vi "test Create Non-default Tag.vi"(8 "error in (no error)":errorcluster, 11 "TestCase in":refnum<class "TagTests.lvclass">) -> (0 "error out":errorcluster, 3 "TestCase out":refnum<class "TagTests.lvclass">)   [LabVIEW 2014, in "TagTests.lvclass"]
uses:
  TagTests.lvclass
  SPLAT/Tag.lvclass
  <vilib>/addons/_JKI Toolkits/VI Tester/TestCase.llb/TestCase.lvclass
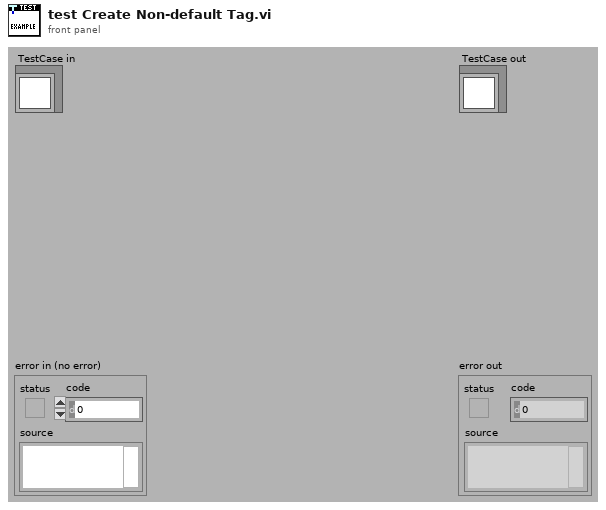
[diagram p1: front panel]
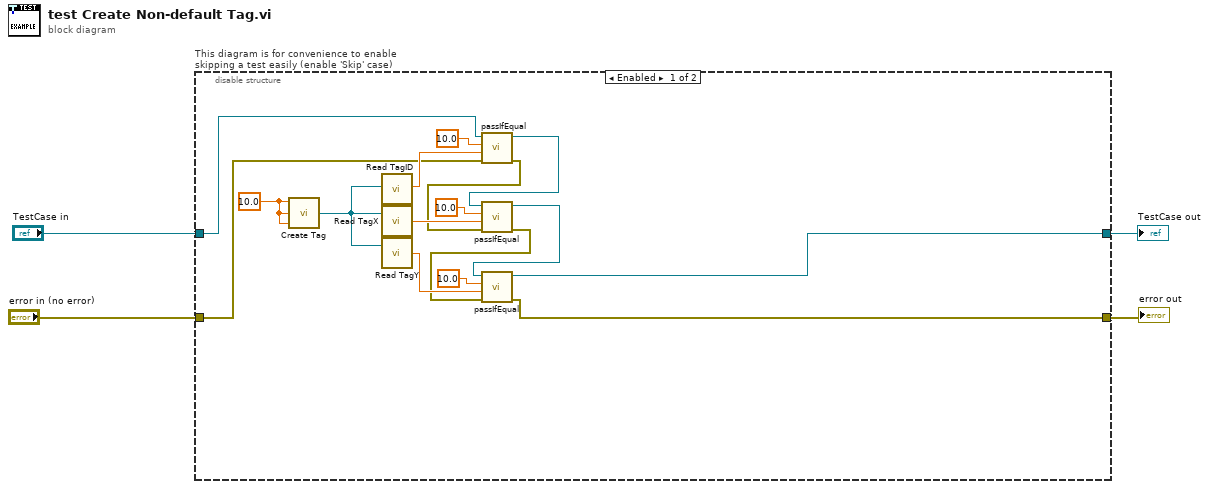
[diagram p0: block diagram]
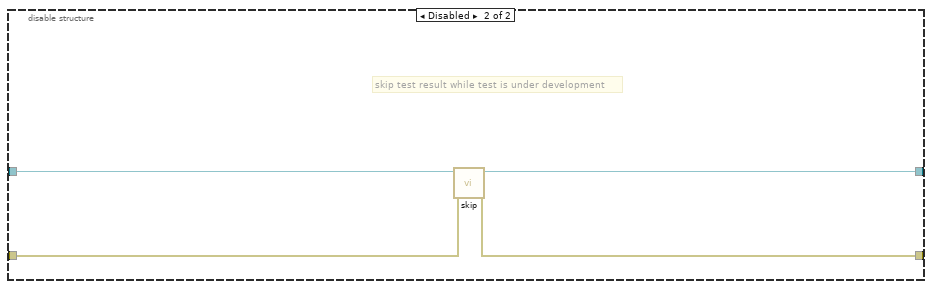
[diagram p2: hidden frame]
diagram:
  n1 = disable-structure "This diagram is for convenience to enable skipping a test easily (enable 'Skip' case)" shown="Enabled" {
    disable-tunnel: "TestCase in" -> [w12 w24]
    disable-tunnel: [w9 w22] -> w1
    disable-tunnel: [w5 w23] -> w3
    disable-tunnel: "error in (no error)" -> [w8 w21]
    frame Enabled {
      w20 = 10.0
      n2 = call "Create Tag.vi"("TagY"=w20, "TagX"=w20, "TagID"=w20) -> ("Tag Out"=w19:refnum<class "Tag.lvclass">)
      n3 = call "Read TagID.vi"("Tag in"=w19) -> ("TagID"=w18:dbl)  [unwired: 16 in, 2 out]
      n4 = call-dynamic "Read TagX.vi"("Tag in"=w19) -> ("RealTagX"=w17:dbl)  [unwired: 1 in, 2 out]
      n5 = call-dynamic "Read TagY.vi"("Tag in"=w19) -> ("RealTagY"=w16:dbl)  [unwired: 1 in, 2 out]
      n6 = call-dynamic "passIfEqual.vi"("error in (no error)"=w8, "y"=w18, "x"=10.0, "TestCase in"=w12) -> ("error out"=w7:errorcluster, "TestCase out"=w11:refnum<class "TagTests.lvclass">)  [unwired: 6 in]
      n7 = call-dynamic "passIfEqual.vi"("error in (no error)"=w7, "y"=w17, "x"=10.0, "TestCase in"=w11) -> ("error out"=w6:errorcluster, "TestCase out"=w10:refnum<class "TagTests.lvclass">)  [unwired: 6 in]
      n8 = call-dynamic "passIfEqual.vi"("error in (no error)"=w6, "y"=w16, "x"=10.0, "TestCase in"=w10) -> ("error out"=w5:errorcluster, "TestCase out"=w9:refnum<class "TagTests.lvclass">)  [unwired: 6 in]
    }
    frame Disabled {
      # "skip test result while test is under development"
      n9 = call <vilib>:"skip.vi"("error in (no error)"=w21, "TestCase in"=w24) -> ("error out"=w23:errorcluster, "TestCase out"=w22:refnum<class "TagTests.lvclass">)  [unwired: 8 in]
    }
  }
  "error out" <- w3
  "TestCase out" <- w1
